vi "Parse Data JSON.vi"(8 "error in (no error)":errorcluster, 10 "JSON String":string, 11 "Identified in":refnum<class "Identified.lvclass">) -> (0 "error out":errorcluster, 1 "Typed?":bool, 2 "Typed Message":refnum<class "Response.lvclass">, 3 "Identified out":refnum<class "Identified.lvclass">)   [LabVIEW 2020, in "obs-websocket.lvlib" / "Identified.lvclass"]
uses:
  Identified.lvclass
  Response/Response.lvclass
  Identified.lvclass/Identified.ctl
  de5579c0-6e0d-4545-abe1-ccd8ba9a1d74.vi
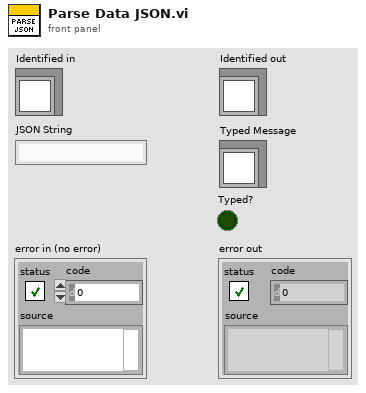
[diagram p1: front panel]
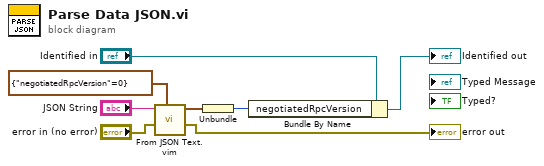
[diagram p0: block diagram]
diagram:
  n1 = call "From JSON Text.vim"("Data Type and Default Value"=cluster{"negotiatedRpcVersion":i32} {"negotiatedRpcVersion"=0}, "error in (no error)"="error in (no error)", "JSON"="JSON String") -> ("error out"=→"error out":errorcluster, "Data out"=w4:cluster{"negotiatedRpcVersion":i32})  [unwired: 7 in]
  n2 = Unbundle(w4) -> ("negotiatedRpcVersion"=w3:i32)
  n3 = Bundle By Name(cluster="Identified in", "negotiatedRpcVersion"=w3) -> (→"Identified out":refnum<class "Identified.lvclass">)
